vi "Calcul CRC.vi"(10 "CRC type":T2(ring), 11 "Trame":string) -> (2 "CRC":string, 3 "Trame + CRC":string)   [LabVIEW 2020, in "Library Commun.lvlib"]
uses:
  Library Commun.lvlib
  Support/AIT - Utility - CRC - CRC Parameters.ctl
  Support/AIT - Utility - CRC - CRC Type.ctl
panel:
  in  "CRC Parameters":T1 {"Final CRC XOR Value" format="%.0x"; "Initial CRC Value" format="%.0x"; "CRC Polynomial" format="%.0x"}
  in  "Trame 2":string
  out "error out":errorcluster caption="sortie d'erreur"
  in  "error in (no error)":errorcluster caption="entrée d'erreur (pas d'erreur)"
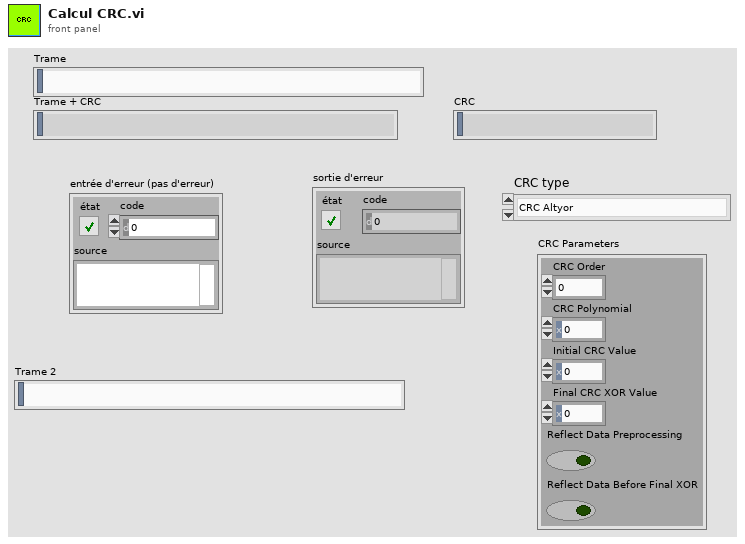
[diagram p1: front panel]
types:
  T1 = typedef "Library Commun.lvlib/AIT - Utility - CRC - CRC Parameters.ctl" = cluster{"CRC Order":u8, "CRC Polynomial":u32, "Initial CRC Value":u32, "Final CRC XOR Value":u32, "Reflect Data Preprocessing":bool, "Reflect Data Before Final XOR":bool}
  T2 = enum16{"CRC Altyor", "CRC Xor On all Bytes", "CRC8", "CRC16", "CRC32", "Other"}
  T3 = typedef "Library Commun.lvlib/AIT - Utility - CRC - CRC Type.ctl" = enum16{"CRC-8", "CRC-16", "CRC-32", "CRC-CCITT", "Other (specify)"}
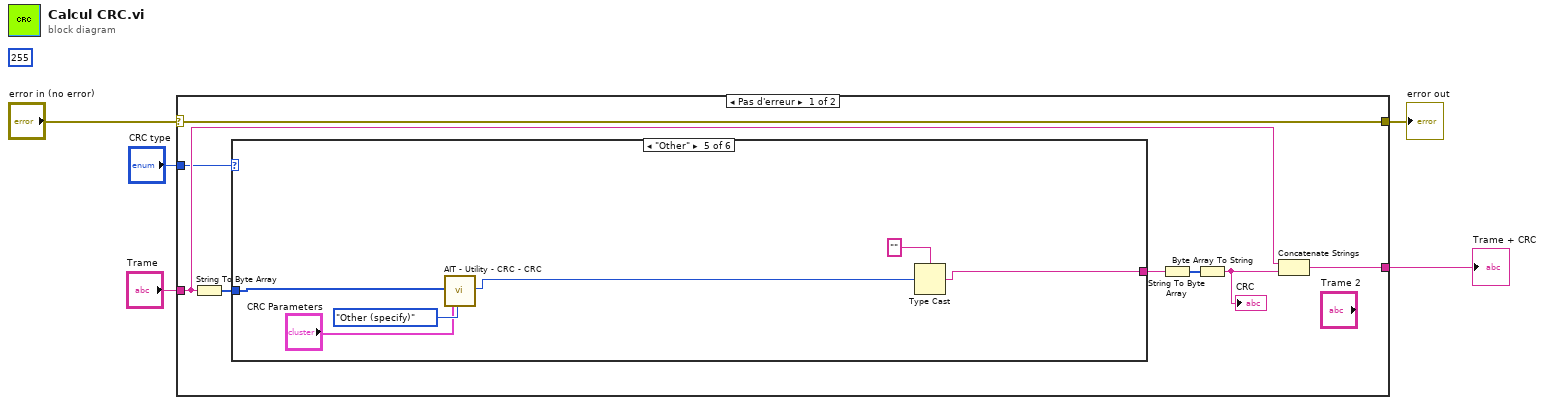
[diagram p0: block diagram]
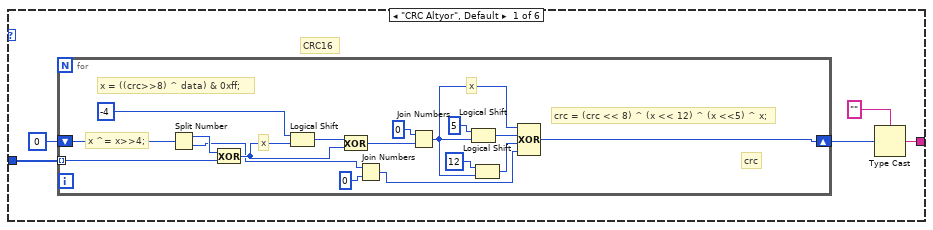
[diagram p2: hidden frame]
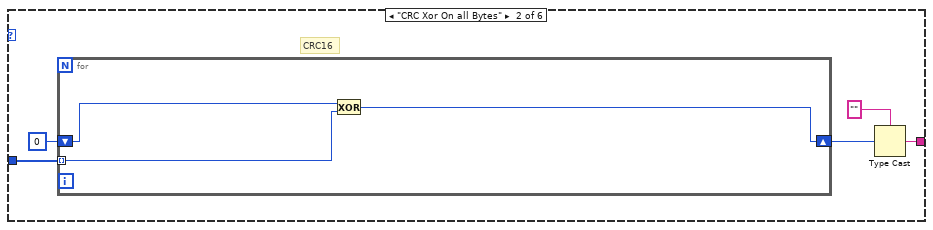
[diagram p3: hidden frame]
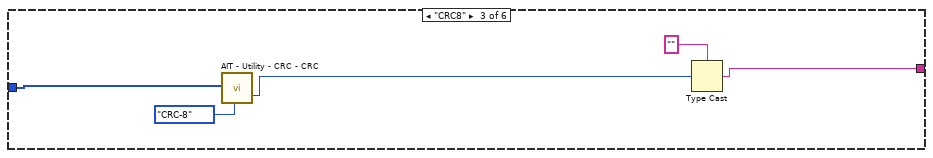
[diagram p4: hidden frame]
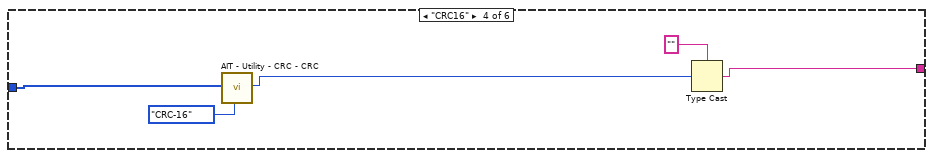
[diagram p5: hidden frame]
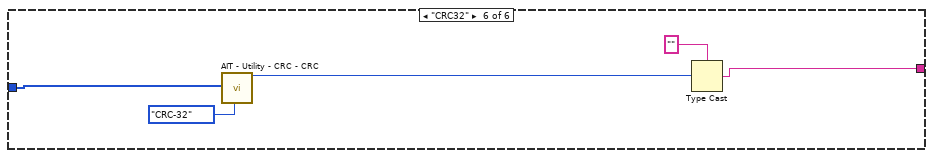
[diagram p6: hidden frame]
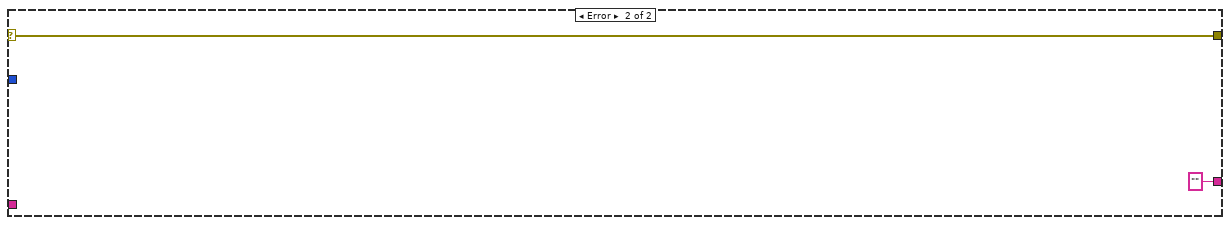
[diagram p7: hidden frame]
diagram:
  (unwired) u8 255 ("x")
  n1 = case shown="Pas d'erreur" "error in (no error)" {
    selector: "error in (no error)" -> [w13 w66]
    tunnel: [w13 w66] -> w4
    tunnel: "Trame" -> [w12 _]
    tunnel: [w11 ""] -> w2
    tunnel: "CRC type" -> [w7 _]
    frame No Error {
      n2 = String To Byte Array(string=w12) -> (unsigned byte array=w6:u8[])
      n3 = case shown="\"Other\"" w7 {
        tunnel: [w16 w38 w45 w51 w57 w62] -> w10
        tunnel: w6 -> [w15 w37 w48 w53 w59 w64]
        frame "CRC Altyor", Default {
          # "CRC16"
          n4 = for {
            tunnel: w15 -> [w29] mode=indexing
            shift-right: [w19] -> w18
            shift-left: u16 0 -> [w28]
            # "crc"
            # "crc = (crc << 8) ^ (x << 12) ^ (x <<5) ^ x;"
            # "x"
            # "x ^= x>>4;"
            # "x"
            # "x = ((crc>>8) ^ data) & 0xff;"
            n5 = Split Number(x=w28) -> (hi(x)=w35:u8, lo(x)=w22:u8)
            n6 = Exclusive Or(1:w29, 2:w35) -> (0:w32:u8)
            n7 = Logical Shift(y=i8 -4, x=w32) -> (x << y=w33:u8)
            n8 = Exclusive Or(1:w32, 2:w33) -> (0:w31:u8)
            n9 = Join Numbers(hi=w22, lo=u8 0) -> ((hi.lo)=w20:u16)
            n10 = Join Numbers(hi=u8 0, lo=w31) -> ((hi.lo)=w24:u16)
            n11 = Logical Shift(y=i8 5, x=w24) -> (x << y=w26:u16)
            n12 = Logical Shift(y=i8 12, x=w24) -> (x << y=w23:u16)
            n13 = Compound Arithmetic op=XOR(w24, w26, w23, w20) -> (w19:u16)
          }
          n14 = Type Cast(type="", x=w18) -> (*(type *) &x=w16:string)
        }
        frame "CRC Xor On all Bytes" {
          # "CRC16"
          n15 = for {
            tunnel: w37 -> [w42] mode=indexing
            shift-right: [w41] -> w40
            shift-left: u8 0 -> [w43]
            n16 = Exclusive Or(1:w42, 2:w43) -> (0:w41:u8)
          }
          n17 = Type Cast(type="", x=w40) -> (*(type *) &x=w38:string)
        }
        frame "CRC8" {
          n18 = call "AIT - Utility - CRC - CRC.vi"("Data Array"=w48, "CRC Calculation"=AIT_-_Utility_-_CRC_-_CRC_Type."CRC-8") -> ("CRC (U8)"=w46:u8)  [unwired: 14 in, 3 out]
          n19 = Type Cast(type="", x=w46) -> (*(type *) &x=w45:string)
        }
        frame "CRC16" {
          n20 = call "AIT - Utility - CRC - CRC.vi"("Data Array"=w53, "CRC Calculation"=AIT_-_Utility_-_CRC_-_CRC_Type."CRC-16") -> ("CRC (U16)"=w49:u16)  [unwired: 14 in, 3 out]
          n21 = Type Cast(type="", x=w49) -> (*(type *) &x=w51:string)
        }
        frame "Other" {
          n22 = call "AIT - Utility - CRC - CRC.vi"("Data Array"=w59, "CRC Parameters"="CRC Parameters", "CRC Calculation"=AIT_-_Utility_-_CRC_-_CRC_Type."Other (specify)") -> ("CRC (U16)"=w55:u16)  [unwired: 13 in, 3 out]
          n23 = Type Cast(type="", x=w55) -> (*(type *) &x=w57:string)
        }
        frame "CRC32" {
          n24 = call "AIT - Utility - CRC - CRC.vi"("Data Array"=w64, "CRC Calculation"=AIT_-_Utility_-_CRC_-_CRC_Type."CRC-32") -> ("CRC (U32)"=w60:u32)  [unwired: 14 in, 3 out]
          n25 = Type Cast(type="", x=w60) -> (*(type *) &x=w62:string)
        }
      }
      n26 = String To Byte Array(string=w10) -> (unsigned byte array=w8:u8[])
      n27 = Byte Array To String(unsigned byte array=w8) -> (string=w9:string)
      "CRC" <- w9
      n28 = Concatenate Strings(w12, w9) -> (w11:string)
    }
    frame Error {
    }
  }
  "error out" <- w4
  "Trame + CRC" <- w2
